vi "GUI_HamamatsuSpectrometer_v1.0.0.vi"() -> ()   [LabVIEW 2013]
uses:
  Shared/MySQL/Preset Query Enum.ctl
  <vilib>/Utility/miscctls.llb/LVOffsetAndMultiplierTypeDef.ctl
  <vilib>/Utility/file.llb/Read From Spreadsheet File (DBL).vi
panel:
  out "FWHM":dbl
  in  "BGlevel":dbl
  out "MeanWavelength":dbl
  out "lambda_r":dbl
  out "lambda_b":dbl
  out "lambda_width (SD)":dbl
  out "AverageCountLevel":dbl
  in  "exposure":dbl
  out "wavelength":dbl[](array[numeric])
  in  "trigger":bool
  in  "save":bool
  out "indecator ref array":refnum<vi>[](array[refnum])
  in  "time to wait (TCP) 2":i32=10
  in  "plot":bool=TRUE
  out "ratio(h)":bool
  out "fixsize":bool
  in  "shotnumber":i32
  out "error (h)":bool
  out "Device Name (h)":string="StagingDG645 1"
  in  "Main Tap":T1(tab)
  out "XY Graph":cluster{"Value":dbl[], "Value":dbl[]}[](graph)
  out "counts":dbl[](array[numeric])
  out "device status::1":string caption="test status"
  out "Intensity Graph 6":dbl[][](graph)
  out "local Port":u16=65427
  out "port or service name":u16=65426
  out "Remote Host":string="192.168.11.97"
  in  "timeout ms (slow resp)":i32=500
  in  "reset":bool
  out "image con closed":bool
  out "image \nconnection":bool
  out "image con closed 2":bool=TRUE
  out "All Devices (h)":string[](array[string])=["StagingDG645 1", "StagingDG645 2"]
  in  "time to wait (TCP)":i32=10
  out "error out":errorcluster
  out "connections (hidden)":variant[](array[variant])=[variant(refnum<k16> refnum), variant(refnum<k16> refnum)]
  in  "time to wait (main loop)":i32=10
  out "Data String":string="Amplitude.Ch AB,3.000000000000\r\nAmplitude.Ch CD,4.000000000000\r\nAmplitude.Ch EF,4.000000000000\r\nAmplitude.Ch GH,4.000000000000\r\nAmplitude.Ch T0,4.000000000000\r\nDelay.Ch A,0.000000000000\r\nDelay.Ch B,0.030000000000\r\nDelay.Ch C,0.000000000000\r\nDelay.Ch D,0.030000000000\r\nDelay.Ch E,0.000000000000\r\nDelay.Ch F,0.030000000000\r\nDelay.Ch G,0.000000000000\r\nDelay.Ch H,0.030000000000\r\nDelay.Ch T0,0.000000000000\r\nDelay.Ch T1,0.030000\r\nInhibit,Triggers\r\nLinked.Ch A,T0\r\nLinked.Ch B,A\r\nLinked.Ch C,T0\r\nLinked.Ch D,C\r\nLinked.Ch E,T0\r\nLinked.Ch F,E\r\nLinked.Ch G,T0\r\nLinked.Ch H,G\r\nLocalSavingPath,c:\\temp\r\nSave,off\r\nTrigger.ExecuteSingleShot,\r\nTrigger.Level,1.000000\r\nTrigger.Rate,10.000000\r\nTrigger.Source,External rising edges\r\ntimeout,0.000000\r\nPolarity.Ch AB,Positive\r\nPolarity.Ch CD,Positive\r\nPolarity.Ch EF,Positive\r\nPolarity.Ch GH,Positive\r\nPolarity.Ch T0,Positive\r\n"
  in  "Local Saving Path":path
  out "error message":string
  out "Data Connection out":bool=TRUE
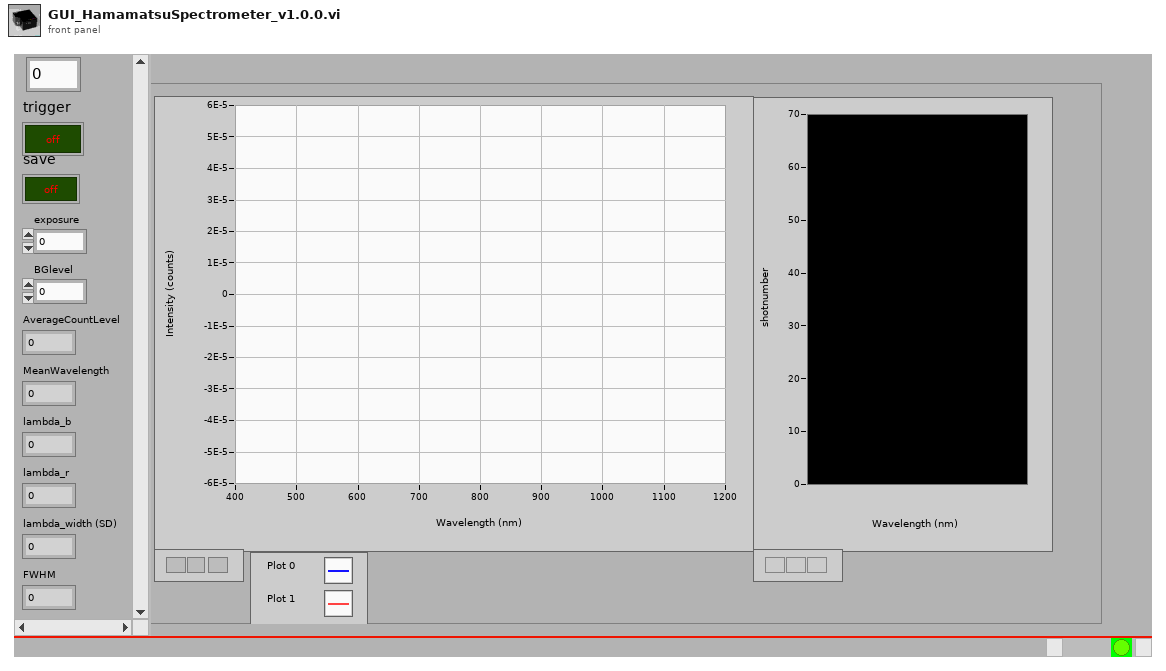
[diagram p1: front panel]
types:
  T1 = enum32{"All Channels", "Network", "Internal", "Advanced"}
  T2 = typedef "Preset Query Enum.ctl" = enum16{"Get Locations", "Get all IPs and MACs", "Get classes", "Get expt variables to set at scanstart for particular device", "Get expt devices and variables with start values", "Get expt devices and variables (with data to get)", "Get expt devices with data to get", "Get Expt devices and GUIs", "Get all devices basic properties", "Get Virtual Devices Core Info", "Get Expt names", "Get experiment basic properties", "Get experiment alarm variables", "Get MC Ports", "Get device network comm port", "Get devicetype lvclass path", "Get basic device properties", "Get Init Order", "Get all setable variables of a device", "Get device variable aliases", "Get force values of all settable variables", "Get all variables of a devicetype", "Get all variables of a device", "Get plotter details", "Get Saved Scans", "Get Scan Info", "GetGeneralGUIs", "Get expt for plotter", "Get plotter IDs from expt", "Get all devices", "Get all Virtual Devices", "Get all aliases", "Get variable and device info for Virtual Device", "GetItemLocatorIP", "Get IPs for GUIs", "Get DeviceType from Device", "GetLocalPortRange", "GetDevicePresetVariables", "Get Device Configuration", "GetAllPresetNames", "GetAllConfigurationNames", "GetPresetDeviceNames"}
  T3 = typedef "LVOffsetAndMultiplierTypeDef.ctl" = cluster{"Offset":dbl, "Multiplier":dbl}
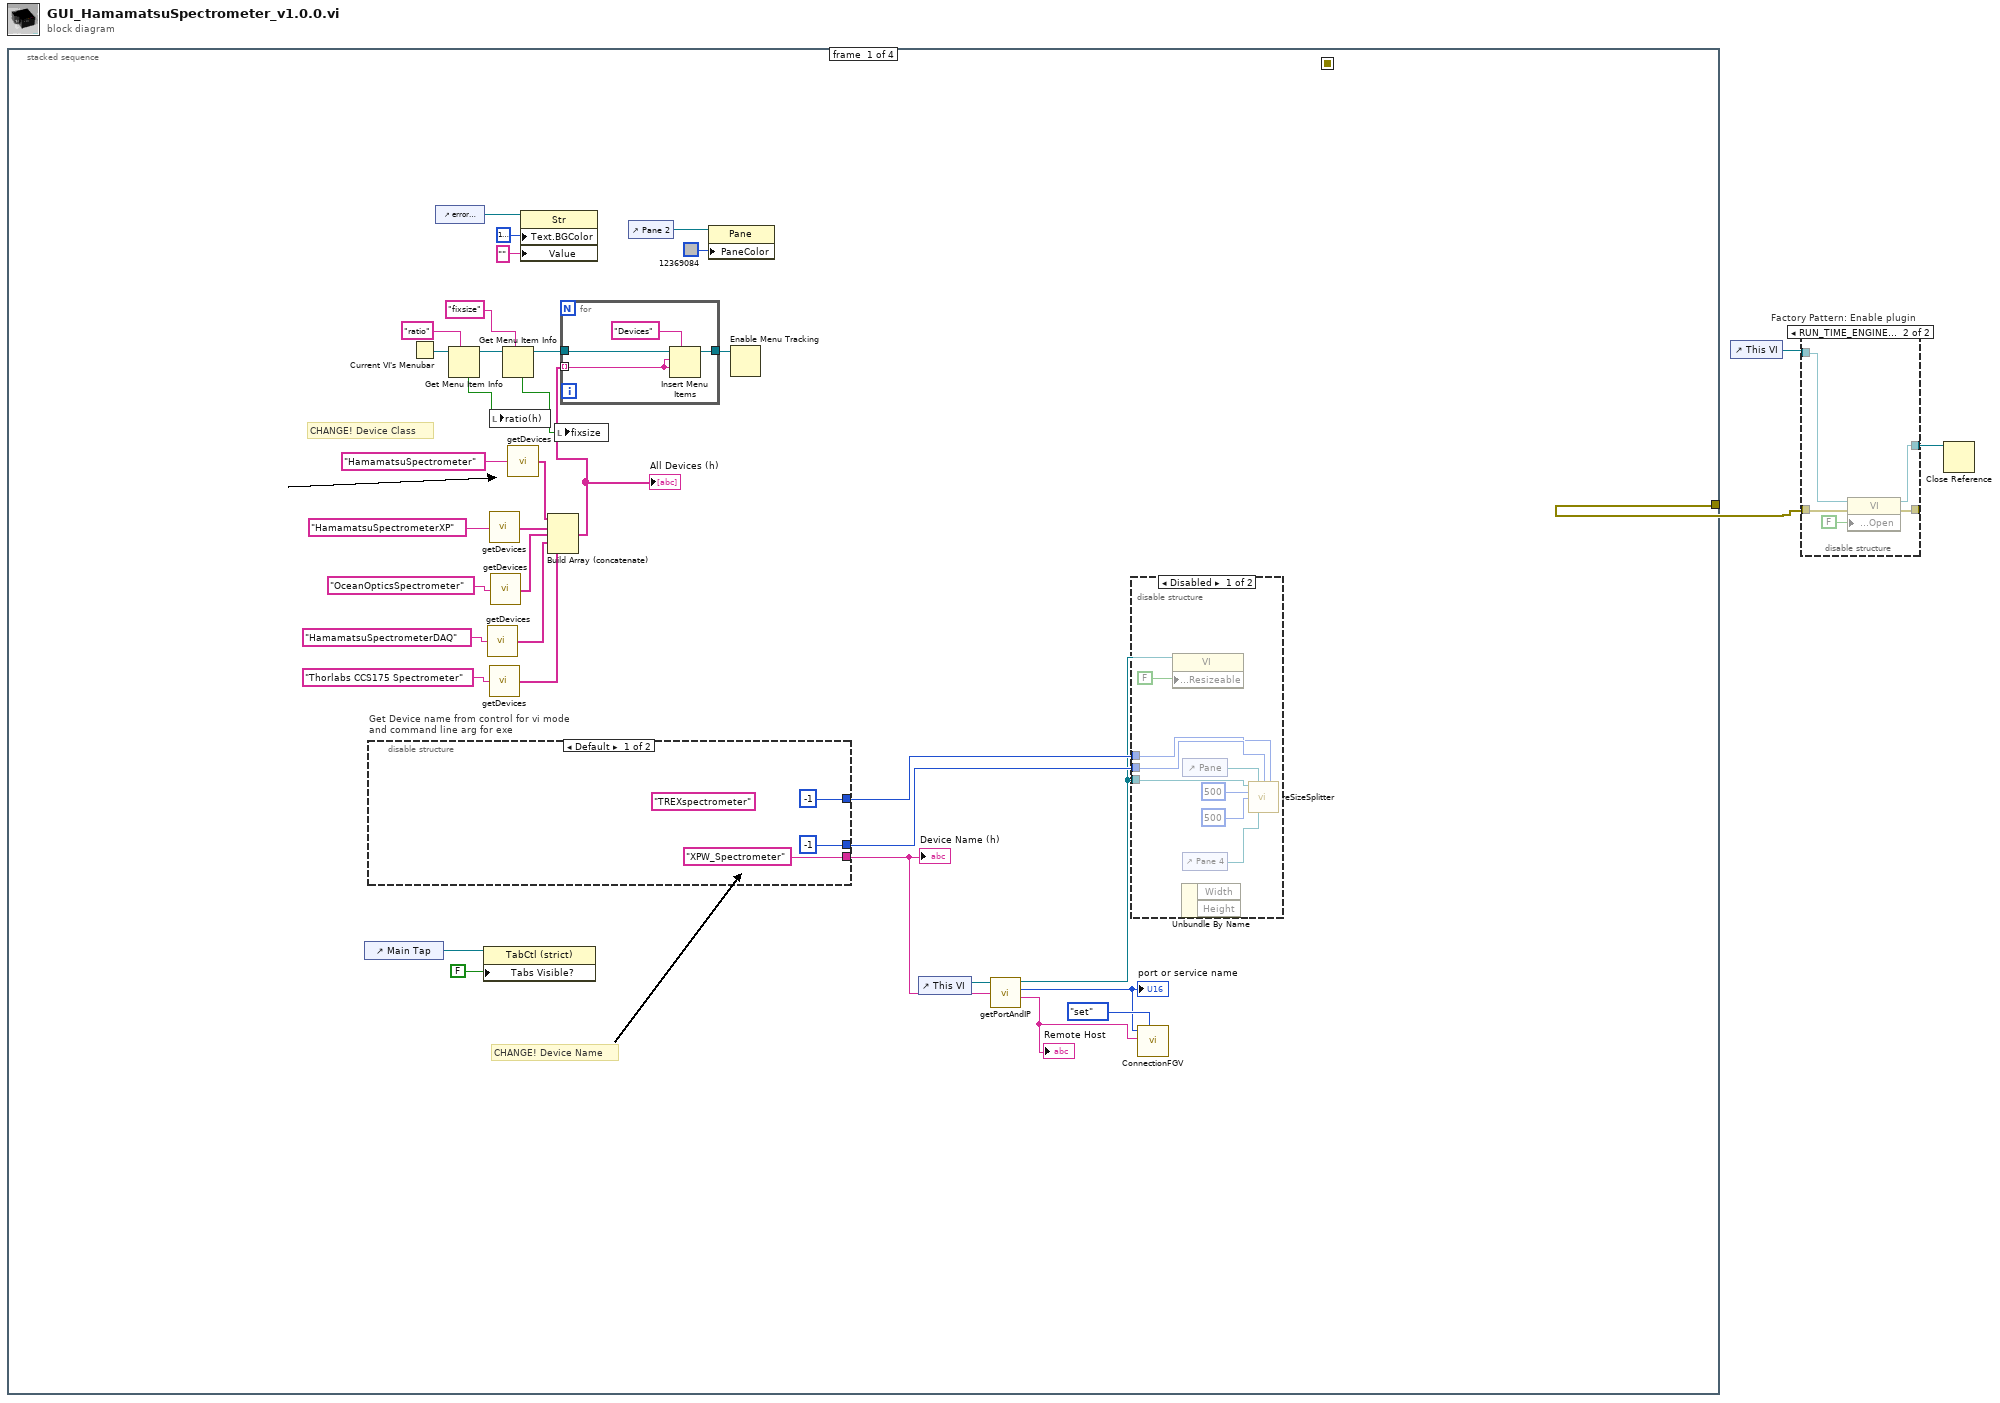
[diagram p0: block diagram]
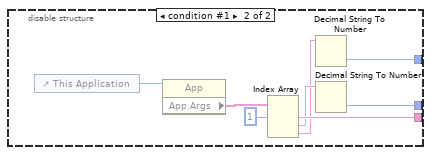
[diagram p4: hidden frame]
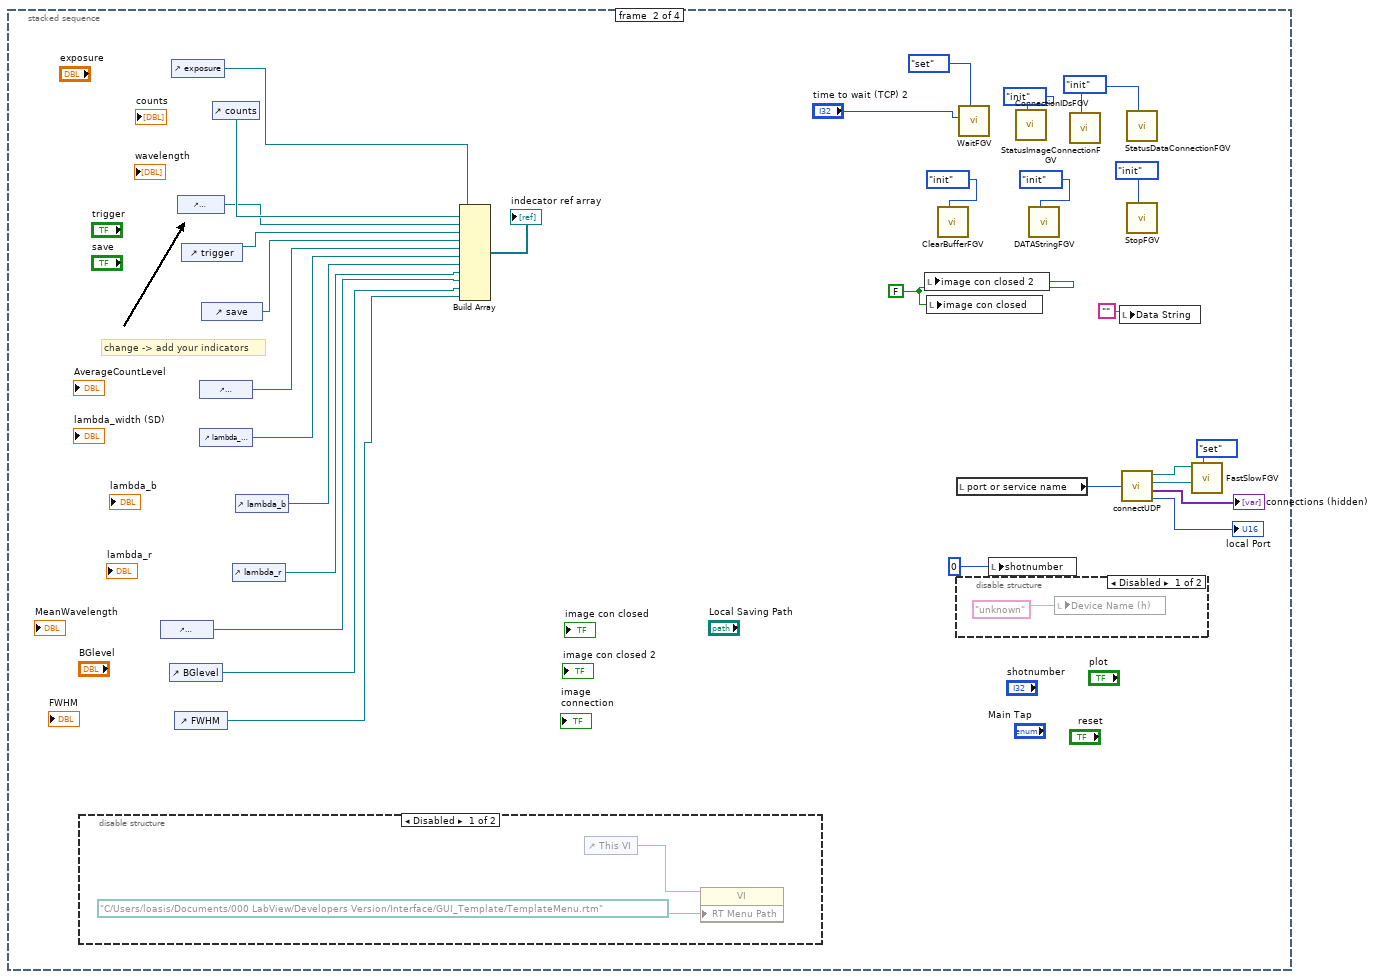
[diagram p5: hidden frame]
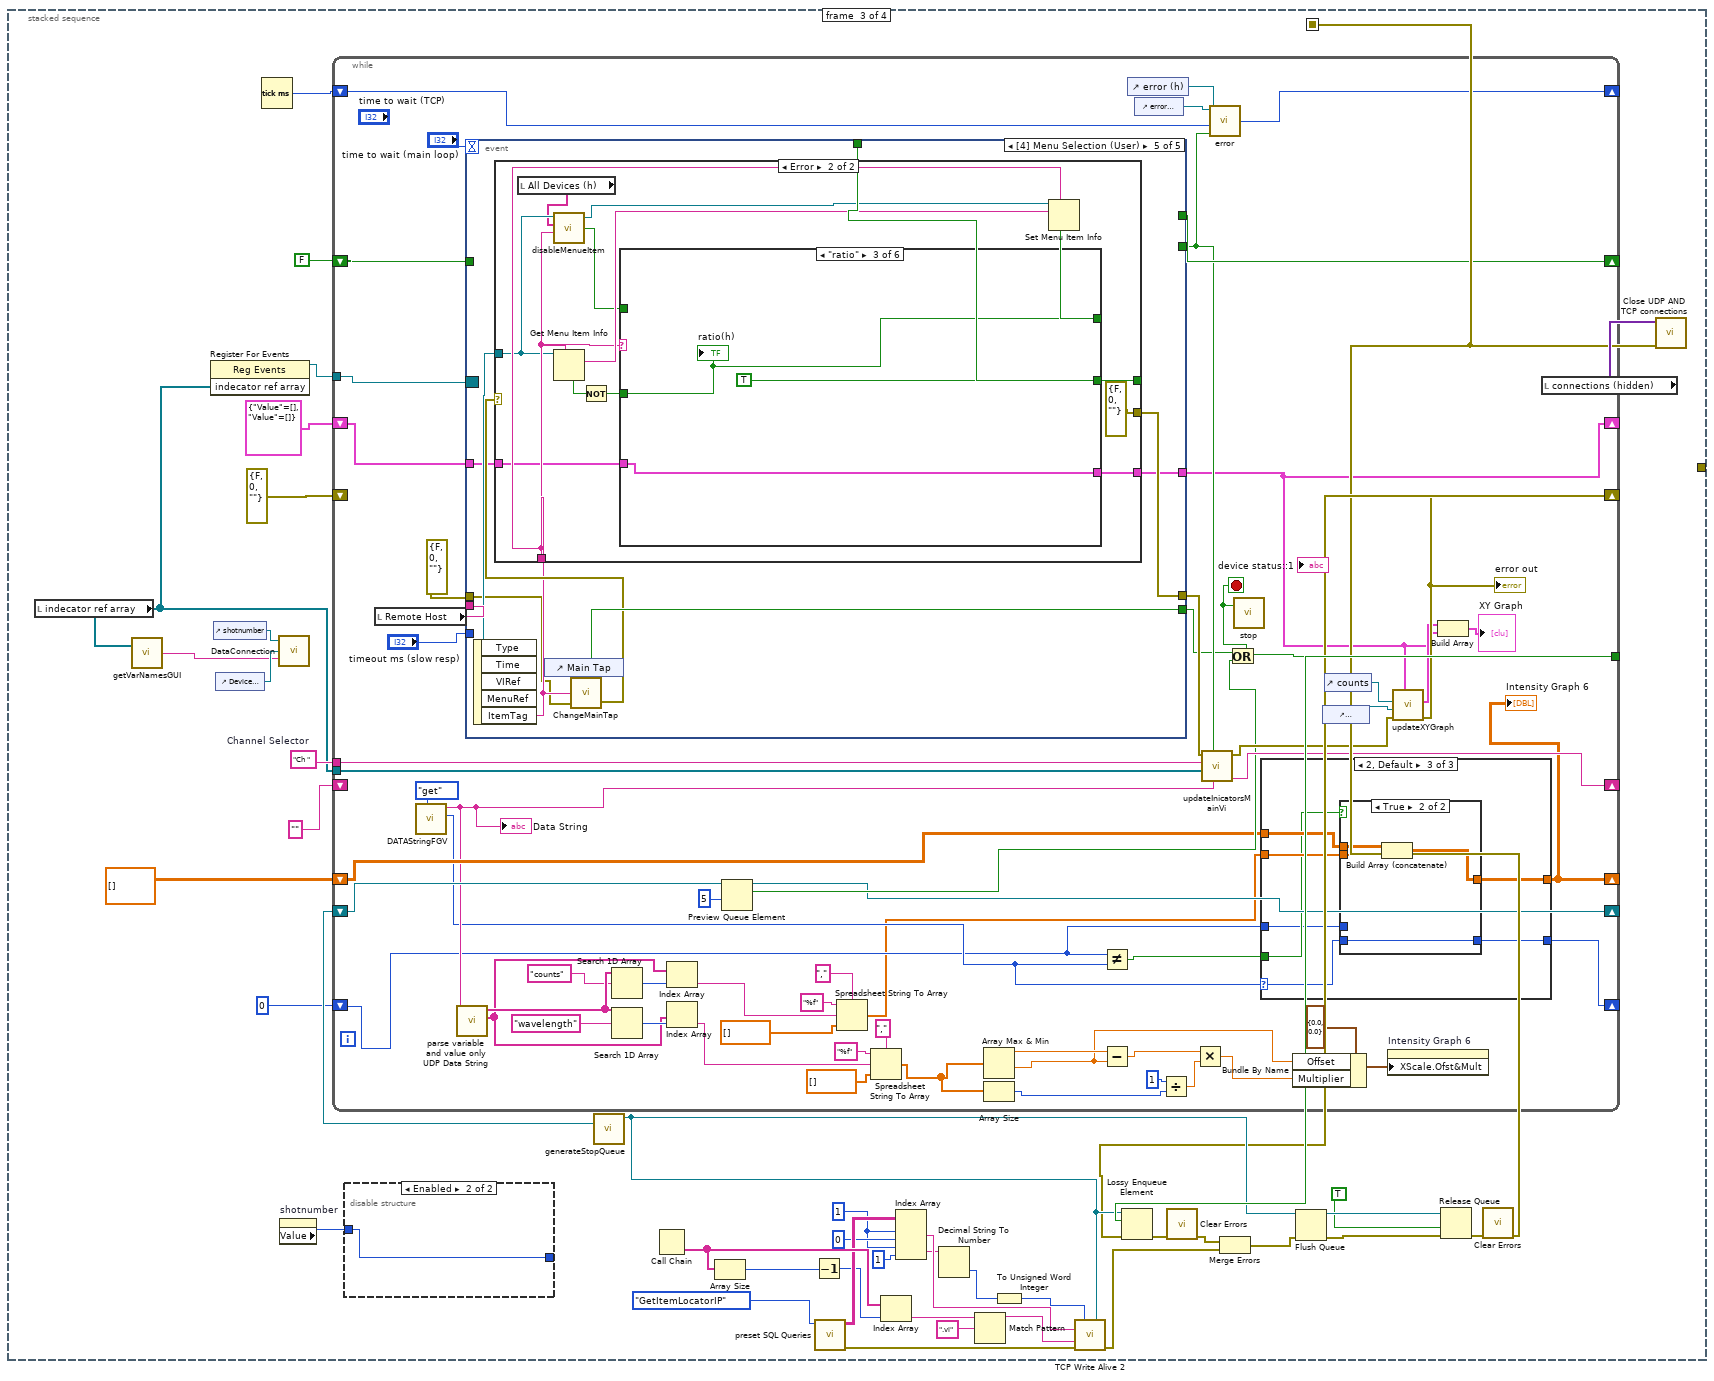
[diagram p8: hidden frame]
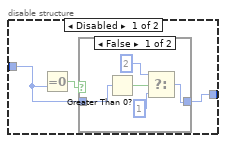
[diagram p9: hidden frame]
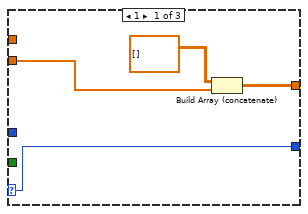
[diagram p11: hidden frame]
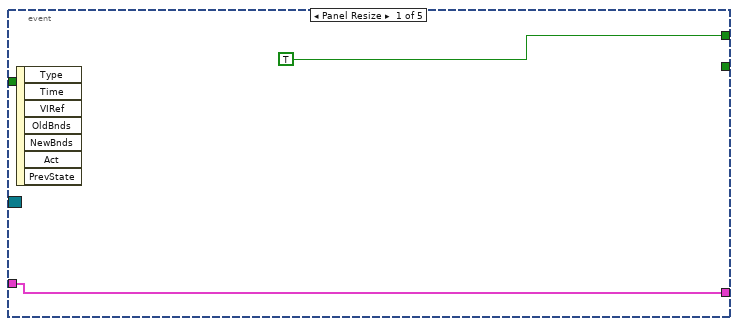
[diagram p14: hidden frame]
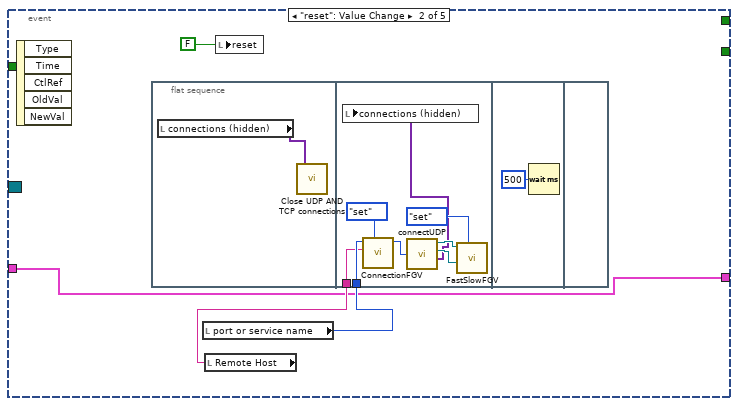
[diagram p15: hidden frame]
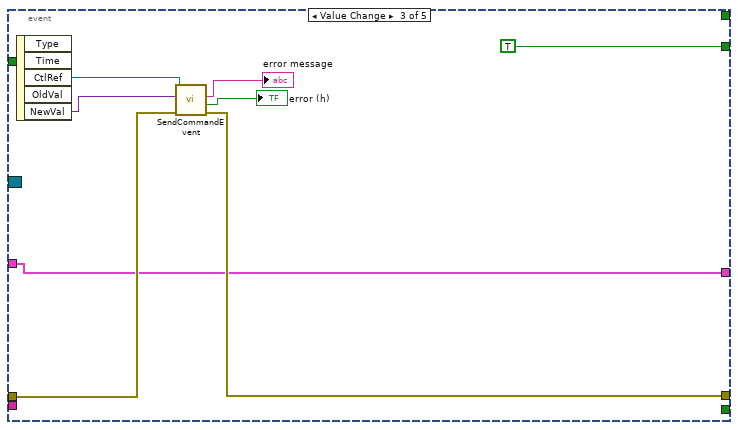
[diagram p16: hidden frame]
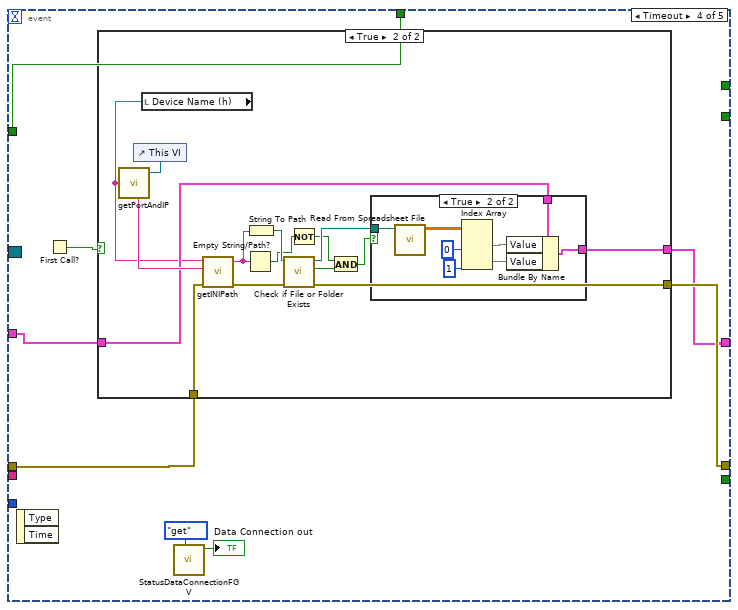
[diagram p17: hidden frame]
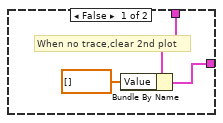
[diagram p19: hidden frame]
diagram:
  n1 = stacked-sequence {
    seq-local: [_ _ w97 _] -> [_ _ _ w368]
    tunnel: [_ _ _ w368] -> w1
    frame #0 {
      # "CHANGE! Device Name"
      # "CHANGE! Device Class"
      n2 = control-ref of="Main Tap"() -> (w38:refnum<vi>)
      n3 = disable-structure "Get Device name from control for vi mode\nand command line arg for exe" shown="Default" {
        disable-tunnel: ["XPW_Spectrometer" ("Device Name for vi mode") w57] -> w34
        disable-tunnel: [i16 -1 ("left") w54] -> w36
        disable-tunnel: [i16 -1 ("left") w53] -> w35
        frame condition #0 (active) {
          (unwired) "TREXspectrometer" ("Device Name for vi mode")
        }
        frame condition #1 {
          n4 = control-ref of="This Application"() -> (w60:refnum<vi>)
          n5 = property class="App"(reference=w60) -> ("App.Args"=w59:string[])  [unwired: 1 in, 2 out]
          n6 = Index Array(array=w59, index #1=1 ("index")) -> (element #1=w57:string, element #2=w56:string, element #3=w55:string)  [unwired: 2 in]
          n7 = Decimal String To Number(string=w55) -> (number=w53:i32)  [unwired: 2 in, 1 out]
          n8 = Decimal String To Number(string=w56) -> (number=w54:i32)  [unwired: 2 in, 1 out]
        }
      }
      "Device Name (h)" <- w34
      n9 = Current VI's Menubar() -> (w26:refnum<k9>)
      n10 = control-ref of="error message"() -> (w20:refnum<vi>)
      n11 = Get Menu Item Info(7:"ratio" ("item tag"), 11:w26) -> (3:w24:refnum<k9>, 4:w25:bool)  [unwired: 1 in, 5 out]
      n12 = property class="TabCtl (strict)"(reference=w38, "Tabs Visible?"=FALSE) -> ()  [unwired: 1 in, 2 out]
      n13 = call "getDevices.vi"("Device Class"="HamamatsuSpectrometerDAQ") -> ("All Devices"=w6:string[])
      n14 = local write "ratio(h)"(w25) -> ()
      n15 = call "getDevices.vi"("Device Class"="HamamatsuSpectrometerXP") -> ("All Devices"=w12:string[])
      n16 = call "getDevices.vi"("Device Class"="Thorlabs CCS175 Spectrometer") -> ("All Devices"=w4:string[])
      n17 = call "getDevices.vi"("Device Class"="OceanOpticsSpectrometer") -> ("All Devices"=w9:string[])
      n18 = Get Menu Item Info(7:"fixsize" ("item tag"), 11:w24) -> (3:w16:refnum<k9>, 4:w22:bool)  [unwired: 1 in, 5 out]
      n19 = call "getDevices.vi"("Device Class"="HamamatsuSpectrometer") -> ("All Devices"=w11:string[])
      n20 = property class="Str"(reference=w20, "Text.BGColor"=u32 16777238, "Value"="") -> ()  [unwired: 1 in, 2 out]
      n21 = Build Array (concatenate)(w11, w12, w9, w6, w4) -> (w10:string[])
      "All Devices (h)" <- w10
      n22 = local write "fixsize"(w22) -> ()
      n23 = for {
        tunnel: w16 -> [w42]
        tunnel: [w41] -> w15
        tunnel: w10 -> [w39] mode=indexing
        n24 = Insert Menu Items(5:"Devices" ("menu tag"), 7:w39, 8:w39, 9:w42) -> (3:w41:refnum<k9>)  [unwired: 2 in, 2 out]
      }
      n25 = control-ref of="Pane 2"() -> (w18:refnum<vi>)
      n26 = property class="Pane"(reference=w18, "PaneColor"=u32 12369084) -> ()  [unwired: 1 in, 2 out]
      n27 = Enable Menu Tracking(4:w15) -> ()  [unwired: 2 in, 2 out]
      n28 = control-ref of="This VI"() -> (w33:refnum<vi>)
      n29 = call "getPortAndIP.vi"("Device Name"=w34, "This Vi"=w33) -> ("Remote Host"=w29:string, "port or service name"=w28:u16, "reference out"=w31:refnum<vi>)  [unwired: 2 in, 2 out]
      "port or service name" <- w28
      "Remote Host" <- w29
      n30 = disable-structure shown="Disabled" {
        disable-tunnel: w36 -> [w48 _]
        disable-tunnel: w35 -> [w47 _]
        disable-tunnel: w31 -> [w45 _]
        frame Disabled {
          n31 = Unbundle By Name() -> ()  [unwired: 1 in, 2 out]
          n32 = control-ref of="Pane"() -> (w49:refnum<vi>)
          n33 = control-ref of="Pane 4"() -> (w46:refnum<vi>)
          n34 = call "reSizeSplitter.vi"("this vi"=w45, "pane"=w49, "left"=w48, "top"=w47, "Width"=u32 500, "Height"=u32 500, "pane2"=w46) -> ()  [unwired: 8 in, 1 out]
        }
        frame Enabled {
        }
      }
      n35 = call "ConnectionFGV.vi"("command"=enum16{"get", "set", "init"}."set", "Remote Host in"=w29, "port or service name in"=w28) -> ()  [unwired: 7 in, 2 out]
      n36 = property class="VI"(reference=w31, "Front Panel.Resizeable"=FALSE ("Front Panel Window:Resizable")) -> ()  [unwired: 1 in, 2 out]
    }
    frame #1 {
      w82 = enum16{"get", "set", "init"}."init" ("Command")
      w88 = FALSE ("new Device Data")
      # "change -> add your indicators"
      n37 = disable-structure shown="Disabled" {
        frame Disabled {
          n38 = control-ref of="This VI"() -> (w92:refnum<vi>)
          n39 = property class="VI"(reference=w92, "RT Menu Path"=path "C:/Users/loasis/Documents/000 LabView/Developers Version/Interface/GUI_Template/TemplateMenu.rtm" ("Run-Time Menu Path")) -> ()  [unwired: 1 in, 2 out]
        }
        frame Enabled {
        }
      }
      n40 = control-ref of="MeanWavelength"() -> (w63:refnum<vi>)
      n41 = control-ref of="BGlevel"() -> (w62:refnum<vi>)
      n42 = control-ref of="exposure"() -> (w68:refnum<vi>)
      n43 = control-ref of="FWHM"() -> (w61:refnum<vi>)
      n44 = control-ref of="wavelength"() -> (w71:refnum<vi>)
      n45 = control-ref of="trigger"() -> (w70:refnum<vi>)
      n46 = control-ref of="AverageCountLevel"() -> (w67:refnum<vi>)
      n47 = control-ref of="lambda_width (SD)"() -> (w66:refnum<vi>)
      n48 = control-ref of="save"() -> (w69:refnum<vi>)
      n49 = control-ref of="counts"() -> (w72:refnum<vi>)
      n50 = control-ref of="lambda_r"() -> (w64:refnum<vi>)
      n51 = control-ref of="lambda_b"() -> (w65:refnum<vi>)
      n52 = Build Array(w68, w72, w71, w70, w69, w67, w66, w65, w64, w63, w62, w61) -> (→"indecator ref array":refnum<vi>[])
      n53 = local write "image con closed 2"(w88) -> ()
      n54 = local write "image con closed"(w88) -> ()
      n55 = call "ClearBufferFGV.vi"("Command"=enum16{"set", "get", "init"}."init") -> ()  [unwired: 10 in, 1 out]
      n56 = local read "port or service name"() -> (w78:u16)
      n57 = disable-structure shown="Disabled" {
        frame Disabled {
          n58 = local write "Device Name (h)"("unknown" ("Device Name")) -> ()
        }
        frame Enabled {
        }
      }
      n59 = call "WaitFGV.vi"("Command"=enum16{"get", "set", "init"}."set", "milliseconds to wait"="time to wait (TCP) 2") -> ()  [unwired: 9 in, 1 out]
      n60 = local write "shotnumber"(0 ("shotnumber")) -> ()
      n61 = call "ConnectionIDsFGV.vi"("Command"=enum16{"add", "get", "init"}."init") -> ()  [unwired: 10 in, 1 out]
      n62 = call "DATAStringFGV.vi"("Command"=enum16{"get", "set", "init"}."init") -> ()  [unwired: 9 in, 2 out]
      n63 = call "StatusImageConnectionFGV.vi"("Command"=w82) -> ()  [unwired: 10 in, 1 out]
      n64 = local write "Data String"("") -> ()
      n65 = call "connectUDP.vi"("port or service name NOT USED"=w78) -> ("fast ID (h)"=w77:refnum<k16>, "slow ID (h)"=w76:refnum<k16>, "connections (hidden)"=→"connections (hidden)":variant[], "local Port"=→"local Port":u16)
      n66 = call "StatusDataConnectionFGV.vi"("Command"=w82) -> ()  [unwired: 10 in, 1 out]
      n67 = call "StopFGV.vi"("Command"=enum16{"set", "get", "init"}."init") -> ()  [unwired: 9 in, 2 out]
      n68 = call "FastSlowFGV.vi"("Command"=enum16{"get", "set", "init"}."set", "slow ID"=w76, "fast ID"=w77) -> ()  [unwired: 7 in, 2 out]
    }
    frame #2 {
      w118 = 1 ("index (row)")
      w127 = "Ch "  # Channel Selector
      n69 = local read "indecator ref array"() -> (w125:refnum<vi>[])
      n70 = call "getVarNamesGUI.vi"("Array"=w125) -> ("String"=w126:string)  [unwired: 1 in]
      n71 = register-events(w125) -> (reference out=w128:refnum<event-registration>)  [unwired: 2 in, 1 out]
      n72 = control-ref of="shotnumber"() -> (w130:refnum<vi>)
      n73 = control-ref of="Device Name (h)"() -> (w129:refnum<vi>)
      n74 = Tick Count (ms)() -> (millisecond timer value=w132:u32)
      n75 = call "DataConnection.vi"("Subscriber list"=w126, "Device Name (h)"=w129, "shotnumber"=w130) -> ()
      n76 = property on="shotnumber" class="DigNum (strict)"() -> ("Value"=w94:i32)  [unwired: 2 in, 2 out]
      n77 = disable-structure shown="Enabled" {
        disable-tunnel: w94 -> [w137 w145]
        disable-tunnel: [w136 w145] -> _
        frame Disabled {
          n78 = Equal To 0?(x=w137) -> (x = 0?=w138:bool)
          n79 = case shown="False" w138 {
            tunnel: w137 -> [w143 w144]
            tunnel: [w139 w144] -> w136
            frame False {
              n80 = Greater Than 0?(x=w143) -> (x > 0?=w142:bool)
              n81 = Select(t=i8 2, s=w142, f=i8 1) -> (s? t:f=w139:i8)
            }
            frame True {
            }
          }
        }
        frame Enabled {
        }
      }
      n82 = call "generateStopQueue.vi"() -> ("STOP Queue out"=w100:refnum<queue>)  [unwired: 10 in, 1 out]
      n83 = while {
        shift-right: [w190] -> w98
        shift-left: errorcluster {"status"=FALSE, "code"=0, "source"=""} ("error out") -> [_]
        tunnel: w125 -> [w199]
        shift-right: [w203] -> _
        shift-left: FALSE -> [w204]
        shift-right: [w202] -> _
        shift-left: w132 -> [w201]
        shift-right: [w194] -> _
        shift-left: "" ("Data String") -> [_]
        tunnel: w128 -> [w197]
        tunnel: w127 -> [w196]
        shift-right: [w184] -> _
        shift-left: w100 -> [w188]
        tunnel: [w185] -> w101
        shift-right: [w182] -> _
        shift-left: dbl[][] [] ("wavelength 2") -> [w183]
        shift-right: [w152] -> _
        shift-left: 0 ("Shot Number") -> [w151]
        shift-right: [w147] -> _
        shift-left: cluster{"Value":dbl[], "Value":dbl[]} {"Value"=[], "Value"=[]} ("reference plot") -> [w149]
        stop <- w185 stop-if-true
        n84 = local read "Remote Host"() -> (w206:string)
        n85 = call "DATAStringFGV.vi"("Command"=enum16{"get", "set", "init"}."get") -> ("Shot Number out"=w154:i32, "Data String out"=w181:string)  [unwired: 9 in]
        "Data String" <- w181
        n86 = call "parse variable and value only UDP Data String.vi"("input string"=w181) -> ("variable values"=w175:string[], "variable names"=w177:string[])  [unwired: 9 in]
        n87 = event shown="[4] Menu Selection (User)" {
          selector: w197 -> [_ _ _ _ _]
          dyn-events: _ -> [_ _ _ _ _]
          timeout: "time to wait (main loop)" -> [_ _ _ _ _]
          tunnel: [_ _ w249 w255 w290] -> w205
          tunnel: w206 -> [_ _ _ _ _]
          tunnel: "timeout ms (slow resp)" -> [_ _ _ _ _]
          tunnel: errorcluster {"status"=FALSE, "code"=0, "source"=""} ("error out") -> [_ _ w246 w256 w291]
          tunnel: [_ _ TRUE _ _] -> w200
          tunnel: [_ _ _ _ w296] -> w187
          tunnel: [_ _ _ w259 w293] -> _
          tunnel: w204 -> [_ _ _ w259 _]
          tunnel: [TRUE _ _ _ _] -> w203
          tunnel: w149 -> [w228 w230 w244 w254 w288]
          tunnel: [w228 w230 w244 w253 w287] -> w147
          event Panel Resize {
            n88 = event-data() -> ()  [unwired: 1 in, 7 out]
          }
          event "reset": Value Change {
            n89 = event-data() -> ()  [unwired: 1 in, 5 out]
            n90 = flat-sequence {
              tunnel: w232 -> [w237]
              tunnel: w231 -> [w236]
              frame #0 {
                n91 = local read "connections (hidden)"() -> (w234:variant[])
                n92 = call "Close UDP AND TCP connections.vi"("appended array"=w234) -> ()  [unwired: 7 in]
              }
              frame #1 {
                n93 = call "ConnectionFGV.vi"("command"=enum16{"get", "set", "init"}."set", "Remote Host in"=w236, "port or service name in"=w237) -> ("port or service name out"=w241:u16)  [unwired: 7 in, 1 out]
                n94 = call "connectUDP.vi"("port or service name NOT USED"=w241) -> ("fast ID (h)"=w240:refnum<k16>, "slow ID (h)"=w239:refnum<k16>, "connections (hidden)"=w235:variant[])  [unwired: 1 out]
                n95 = local write "connections (hidden)"(w235) -> ()
                n96 = call "FastSlowFGV.vi"("Command"=enum16{"get", "set", "init"}."set", "slow ID"=w239, "fast ID"=w240) -> ()  [unwired: 7 in, 2 out]
              }
              frame #2 {
                n97 = Wait (ms)(milliseconds to wait=u32 500) -> ()  [unwired: 1 out]
              }
              frame #3 {
              }
            }
            n98 = local read "port or service name"() -> (w232:u16)
            n99 = local read "Remote Host"() -> (w231:string)
            n100 = local write "reset"(FALSE ("reset")) -> ()
          }
          event Value Change {
            n101 = event-data() -> ("CtlRef"=w251:refnum<vi>, "NewVal"=w250:variant)  [unwired: 1 in, 3 out]
            n102 = call "SendCommandEvent.vi"("error out 2"=w246, "NewVal"=w250, "CtlRef"=w251) -> ("error out"=w249:errorcluster, "error (h)"=→"error (h)":bool, "error message"=→"error message":string)  [unwired: 5 in, 1 out]
          }
          event Timeout {
            n103 = event-data() -> ()  [unwired: 1 in, 2 out]
            n104 = First Call?() -> (First Call?: T/F=w252:bool)
            n105 = case shown="True" w252 {
              tunnel: w256 -> [w260 w266]
              tunnel: [w260 w265] -> w255
              tunnel: w254 -> [w261 w264]
              tunnel: [w261 w263] -> w253
              frame False {
              }
              frame True {
                n106 = control-ref of="This VI"() -> (w275:refnum<vi>)
                n107 = local read "Device Name (h)"() -> (w262:string)
                n108 = call "getPortAndIP.vi"("Device Name"=w262, "This Vi"=w275) -> ("Device Type"=w267:string)  [unwired: 2 in, 4 out]
                n109 = call "getINIPath.vi"("error in (no error)"=w266, "DeviceType Name"=w267, "Device Name"=w262) -> ("error out"=w265:errorcluster, "reference trace path"=w274:string)  [unwired: 7 in]
                n110 = Empty String/Path?(string/path=w274) -> (empty?=w271:bool)
                n111 = String To Path(string=w274) -> (path=w273:path)
                n112 = call <vilib>:"Check if File or Folder Exists.vi"("path"=w273) -> ("file or folder exists?"=w269:bool, "dup path"=w272:path)  [unwired: 8 in, 1 out]
                n113 = Not(x=w271) -> (.not. x?=w270:bool)
                n114 = And(x=w270, y=w269) -> (x .and. y?=w268:bool)
                n115 = case shown="True" w268 {
                  tunnel: w264 -> [w278 w286]
                  tunnel: [w277 w280] -> w263
                  tunnel: w272 -> [_ w279]
                  frame False {
                    # "When no trace,clear 2nd plot"
                    n116 = Bundle By Name(cluster=w278, "Value"=dbl[] []) -> (w277:cluster{"Value":dbl[], "Value":dbl[]})
                  }
                  frame True {
                    n117 = call-poly <vilib>:"Read From Spreadsheet File.vi"("file path (dialog if empty)"=w279) -> ("all rows"=w285:dbl[][])  [unwired: 6 in, 4 out]
                    n118 = Index Array(array=w285, index (col) #1=0 ("disabled index (col)"), index (col) #2=1 ("index (col)")) -> (element #1=w282:dbl[], element #2=w281:dbl[])  [unwired: 2 in]
                    n119 = Bundle By Name(cluster=w286, "Value"=w282, "Value"=w281) -> (w280:cluster{"Value":dbl[], "Value":dbl[]})
                  }
                }
              }
            }
            n120 = call "StatusDataConnectionFGV.vi"("Command"=enum16{"get", "set", "init"}."get") -> ("Data Connection out"=→"Data Connection out":bool)  [unwired: 10 in]
          }
          event Menu Selection (User) {
            n121 = event-data() -> ("MenuRef"=w292:refnum<k9>, "ItemTag"=w294:string)  [unwired: 1 in, 3 out]
            n122 = control-ref of="Main Tap"() -> (w289:refnum<vi>)
            n123 = call "ChangeMainTap.vi"("error in"=w291, "ItemTag"=w294, "reference"=w289) -> ("error out"=w295:errorcluster, "Boolean"=w296:bool)
            n124 = case shown="Error" w295 {
              selector: w295 -> [w298 _]
              tunnel: w292 -> [_ w306]
              tunnel: [_ w308] -> w293
              tunnel: w294 -> [_ w307]
              tunnel: [w298 errorcluster {"status"=FALSE, "code"=0, "source"=""} ("error IO")] -> w290
              tunnel: w288 -> [w297 w300]
              tunnel: [w297 w299] -> w287
              frame No Error {
              }
              frame Error {
                n125 = local read "All Devices (h)"() -> (w301:string[])
                n126 = call "disableMenueItem.vi"("ItemTag"=w307, "All Devices (h)"=w301, "MenuRef"=w306) -> ("this is a Device(tag)"=w305:bool, "menu reference out"=w304:refnum<k9>)  [unwired: 1 in, 1 out]
                n127 = Get Menu Item Info(7:w307, 11:w306) -> (2:w310:string, 4:w311:bool)  [unwired: 1 in, 5 out]
                n128 = Not(x=w311) -> (.not. x?=w309:bool)
                n129 = case shown="\"ratio\"" w307 {
                  selector: w307 -> [_ w320 _ _ _ _]
                  tunnel: w309 -> [w313 w318 w352 _ _ _]
                  tunnel: [_ _ TRUE _ _ _] -> w308
                  tunnel: w305 -> [_ w321 _ _ _ _]
                  tunnel: [w313 w319 w352 _ _ _] -> w303
                  tunnel: w300 -> [w312 w317 w351 w354 w362 w365]
                  tunnel: [w312 w316 w351 w354 w362 w365] -> w299
                  frame "fixsize" {
                    n130 = control-ref of="This VI"() -> (w315:refnum<vi>)
                    n131 = Not(x=w313) -> (.not. x?=w314:bool)
                    n132 = property class="VI"(reference=w315, "Front Panel.Resizeable"=w314) -> ()  [unwired: 1 in, 2 out]
                    "fixsize" <- w313
                  }
                  frame Default {
                    n133 = case shown="True" w321 {
                      tunnel: w320 -> [_ w323]
                      tunnel: [_ w334] -> w319
                      tunnel: w318 -> [_ w334]
                      tunnel: w317 -> [w322 w333]
                      tunnel: [w322 w332] -> w316
                      frame False {
                      }
                      frame True {
                        n134 = control-ref of="This VI"() -> (w339:refnum<vi>)
                        n135 = call "getPortAndIP.vi"("Device Name"=w323, "This Vi"=w339) -> ("Device Type"=w331:string, "Remote Host"=w338:string, "port or service name"=w337:u16)  [unwired: 2 in, 2 out]
                        n136 = call "getINIPath.vi"("DeviceType Name"=w331, "Device Name"=w323) -> ("reference trace path"=w330:string)  [unwired: 8 in, 1 out]
                        n137 = local write "Remote Host"(w338) -> ()
                        n138 = local write "port or service name"(w337) -> ()
                        n139 = Empty String/Path?(string/path=w330) -> (empty?=w327:bool)
                        n140 = String To Path(string=w330) -> (path=w329:path)
                        n141 = call <vilib>:"Check if File or Folder Exists.vi"("path"=w329) -> ("file or folder exists?"=w325:bool, "dup path"=w328:path)  [unwired: 8 in, 1 out]
                        n142 = Not(x=w327) -> (.not. x?=w326:bool)
                        n143 = And(x=w326, y=w325) -> (x .and. y?=w324:bool)
                        n144 = control-ref of="reset"() -> (w336:refnum<vi>)
                        n145 = case shown="True" w324 {
                          tunnel: w333 -> [w342 w350]
                          tunnel: [w341 w344] -> w332
                          tunnel: w328 -> [_ w343]
                          frame False {
                            # "When no trace,clear 2nd plot"
                            n146 = Bundle By Name(cluster=w342, "Value"=dbl[] []) -> (w341:cluster{"Value":dbl[], "Value":dbl[]})
                          }
                          frame True {
                            n147 = call-poly <vilib>:"Read From Spreadsheet File.vi"("file path (dialog if empty)"=w343) -> ("all rows"=w349:dbl[][])  [unwired: 6 in, 4 out]
                            n148 = Index Array(array=w349, index (col) #1=0 ("disabled index (col)"), index (col) #2=1 ("index (col)")) -> (element #1=w346:dbl[], element #2=w345:dbl[])  [unwired: 2 in]
                            n149 = Bundle By Name(cluster=w350, "Value"=w346, "Value"=w345) -> (w344:cluster{"Value":dbl[], "Value":dbl[]})
                          }
                        }
                        n150 = property class="Bool (strict)"(reference=w336, "Val(Sgnl)"=TRUE ("Value (Signaling)")) -> ()  [unwired: 1 in, 2 out]
                      }
                    }
                  }
                  frame "ratio" {
                    "ratio(h)" <- w352
                  }
                  frame "Local Saving Path" {
                    n151 = control-ref of="Local Saving Path"() -> (w355:refnum<vi>)
                    n152 = property class="Path"(reference=w355) -> (reference out=w358:refnum<vi>, "Value"=w359:path)  [unwired: 1 in, 1 out]
                    n153 = call "changePath.vi"("Local Saving in (h)"=w359) -> ("change (h)"=w357:bool, "Local Saving out (h)"=w356:path)  [unwired: 9 in]
                    n154 = case shown="True" w357 {
                      tunnel: w358 -> [_ w361]
                      tunnel: w356 -> [_ w360]
                      frame False {
                      }
                      frame True {
                        n155 = property class="Path"(reference=w361, "Val(Sgnl)"=w360) -> ()  [unwired: 1 in, 2 out]
                      }
                    }
                  }
                  frame "reset" {
                    n156 = control-ref of="reset"() -> (w364:refnum<vi>)
                    n157 = property class="Bool (strict)"(reference=w364, "Val(Sgnl)"=TRUE ("Value (Signaling)")) -> ()  [unwired: 1 in, 2 out]
                  }
                  frame "clear" {
                    n158 = control-ref of="reset"() -> (w367:refnum<vi>)
                    n159 = property class="Bool (strict)"(reference=w367, "Val(Sgnl)"=TRUE ("Value (Signaling)")) -> ()  [unwired: 1 in, 2 out]
                  }
                }
                n160 = Set Menu Item Info(6:w303, 7:w307, 10:w310, 11:w304) -> ()  [unwired: 3 in, 2 out]
              }
            }
          }
        }
        n161 = Search 1D Array(1D array=w177, element="counts") -> (index of element=w176:i32)  [unwired: 1 in]
        n162 = Search 1D Array(1D array=w177, element="wavelength") -> (index of element=w179:i32)  [unwired: 1 in]
        n163 = Index Array(array=w175, index=w176) -> (element=w170:string)
        n164 = Index Array(array=w175, index=w179) -> (element=w165:string)
        n165 = Preview Queue Element ("get stop queue value")(queue=w188, timeout in ms (-1)=5) -> (queue out=w184:refnum<queue>, element=w186:bool)  [unwired: 1 in, 2 out]
        n166 = Spreadsheet String To Array(delimiter (Tab)=",", format string="%f", spreadsheet string=w170, array type (2D Dbl)=dbl[] []) -> (array=w150:dbl[])
        n167 = Spreadsheet String To Array(delimiter (Tab)=",", format string="%f", spreadsheet string=w165, array type (2D Dbl)=dbl[] []) -> (array=w164:dbl[])
        n168 = Array Max & Min(array=w164) -> (max value=w161:dbl, min value=w156:dbl)  [unwired: 2 out]
        n169 = Array Size(array=w164) -> (size(s)=w163:i32)
        n170 = Not Equal?(x=w151, y=w154) -> (x != y?=w153:bool)
        n171 = Subtract(x=w161, y=w156) -> (x-y=w160:dbl)
        n172 = control-ref of="error (h)"() -> (w192:refnum<vi>)
        n173 = control-ref of="error message"() -> (w193:refnum<vi>)
        n174 = Divide(x=1, y=w163) -> (x/y=w159:dbl)
        n175 = Multiply(x=w160, y=w159) -> (x*y=w155:dbl)
        n176 = call "updateInicatorsMainVi.vi"("Data String out"=w181, "Boolean"=w200, "Array"=w199, "Channel Selector"=w196, "error in"=w205) -> ("Data String out 2"=w194:string, "error out"=w191:errorcluster)  [unwired: 4 in, 1 out]
        n177 = call "error.vi"("Boolean"=w200, "millisecond timer value"=w201, "reference"=w192, "error message"=w193) -> ("millisecond timer value 2"=w202:u32)
        n178 = Or(x=w187, y=w186) -> (x .or. y?=w185:bool)
        n179 = call "stop.vi"("Boolean"=w185) -> ()
        n180 = case shown="2, Default" w154 {
          selector: w154 -> [w209 w213 w217]
          tunnel: w183 -> [_ w214 w221]
          tunnel: w150 -> [w211 _ w220]
          tunnel: [w210 w214 w219] -> w182
          tunnel: w153 -> [_ _ w218]
          tunnel: [w209 w213 w216] -> w152
          tunnel: w151 -> [_ _ w215]
          frame 1 {
            n181 = Build Array (concatenate)(dbl[][] [] ("wavelength 2"), w211) -> (w210:dbl[][])
          }
          frame 0 {
          }
          frame 2, Default {
            n182 = case shown="True" w218 {
              tunnel: w221 -> [w223 w227]
              tunnel: [w223 w226] -> w219
              tunnel: w220 -> [_ w225]
              tunnel: w217 -> [_ w224]
              tunnel: [w222 w224] -> w216
              tunnel: w215 -> [w222 _]
              frame False {
              }
              frame True {
                n183 = Build Array (concatenate)(w227, w225) -> (w226:dbl[][])
              }
            }
          }
        }
        "Intensity Graph 6" <- w182
        n184 = Bundle By Name(cluster=T3 {"Offset"=0.0, "Multiplier"=0.0} ("X Scale.Offset and Multiplier"), "Offset"=w156, "Multiplier"=w155) -> (w157:T3)
        n185 = control-ref of="wavelength"() -> (w178:refnum<vi>)
        n186 = control-ref of="counts"() -> (w180:refnum<vi>)
        n187 = property on="Intensity Graph 6" class="IntGraph (strict)"("XScale.Ofst&Mult"=w157) -> ()  [unwired: 2 in, 2 out]
        n188 = call "updateXYGraph.vi"("reference plot"=w147, "error in (no error)"=w191, "wavelength"=w178, "counts"=w180) -> ("error out"=w190:errorcluster, "output cluster"=w148:cluster{"Value":dbl[], "Value":dbl[]})  [unwired: 6 in]
        "error out" <- w190
        n189 = Build Array(w148, w147) -> (→"XY Graph":cluster{"Value":dbl[], "Value":dbl[]}[])
      }
      n190 = Call Chain() -> (call chain=w124:string[])
      n191 = Array Size(array=w124) -> (size(s)=w109:i32)
      n192 = Decrement(x=w109) -> (x-1=w110:i32)
      n193 = call "preset SQL Queries.vi"("Preset Query"=Preset_Query_Enum."GetItemLocatorIP") -> ("error out"=w115:errorcluster, "data"=w121:string[][])  [unwired: 8 in, 1 out]
      n194 = Index Array(array=w124, index=w110) -> (element=w111:string)
      n195 = Index Array(array=w121, index (row) #1=w118, index (col) #1=0 ("disabled index (col)"), index (row) #2=w118, index (col) #2=1 ("disabled index (col)")) -> (element #1=w123:string, element #2=w122:string)
      n196 = Decimal String To Number(string=w122) -> (number=w116:i32)  [unwired: 2 in, 1 out]
      n197 = Match Pattern(string=w111, regular expression=".vi") -> (before substring=w113:string)  [unwired: 1 in, 3 out]
      n198 = To Unsigned Word Integer(number=w116) -> (unsigned 16bit integer=w117:u16)
      n199 = call "TCP Write Alive 2.vi"("MultiCast Port"=w117, "Stopqueue"=w100, "address"=w123, "Name"=w113, "error in (no error)"=w115) -> ("error out"=w99:errorcluster)  [unwired: 8 in, 2 out]
      n200 = Lossy Enqueue Element(queue=w100, element=w101, error in (no error)=w98) -> (error out=w102:errorcluster)  [unwired: 3 out]
      n201 = call <vilib>:"Clear Errors.vi"("error in (no error)"=w102) -> ("error out"=w103:errorcluster)  [unwired: 6 in]
      n202 = Merge Errors(w103, w99) -> (w107:errorcluster)
      n203 = Flush Queue(queue=w100, error in (no error)=w107) -> (queue out=w108:refnum<queue>, error out=w104:errorcluster)  [unwired: 1 out]
      n204 = Release Queue(queue=w108, force destroy? (F)=TRUE, error in (no error)=w104) -> (error out=w106:errorcluster)  [unwired: 2 out]
      n205 = call <vilib>:"Clear Errors.vi"("error in (no error)"=w106) -> ("error out"=w97:errorcluster)  [unwired: 6 in]
      n206 = local read "connections (hidden)"() -> (w134:variant[])
      n207 = call "Close UDP AND TCP connections.vi"("error in"=w97, "appended array"=w134) -> ()  [unwired: 6 in]
    }
    frame #3 {
      n208 = control-ref of="Main  Control"() -> (w370:refnum<vi>)
      n209 = property class="TabCtl (strict)"(reference=w370, "Tabs Visible?"=TRUE) -> ()  [unwired: 1 in, 2 out]
      n210 = property class="TabCtl (strict)"(reference=w370, "Tab Location"=enum32{"Top", "Bottom", "Left", "Right"}."Bottom") -> ()  [unwired: 1 in, 2 out]
      n211 = flat-sequence {
        frame #0 {
          n212 = Wait (ms)(milliseconds to wait=u32 0) -> ()  [unwired: 1 out]
        }
        frame #1 {
        }
        frame #2 {
          n213 = disable-structure shown="Disabled" {
            frame Disabled {
              n214 = control-ref of="This VI"() -> (w375:refnum<vi>)
              n215 = case shown="True" FALSE {
                tunnel: w375 -> [w376 w379]
                tunnel: [w376 w377] -> w374
                frame False {
                }
                frame True {
                  n216 = property class="VI" props=["Front Panel.Open"](reference=w379) -> (reference out=w378:refnum<vi>)  [unwired: 1 in, 2 out]
                  n217 = invoke class="VI" method="FP.Close"(reference=w378) -> (reference out=w377:refnum<vi>)  [unwired: 2 in, 2 out]
                }
              }
              n218 = Close Reference(reference=w374) -> ()  [unwired: 1 in, 1 out]
            }
            frame Enabled {
            }
          }
        }
      }
    }
  }
  n219 = control-ref of="This VI"() -> (w2:refnum<vi>)
  n220 = disable-structure "Factory Pattern: Enable plugin" shown="RUN_TIME_ENGINE==True" {
    disable-tunnel: w1 -> [_ w384]
    disable-tunnel: w2 -> [w380 w383]
    disable-tunnel: [_ w382] -> _
    disable-tunnel: [w380 w381] -> w3
    frame condition #0 (active) {
    }
    frame condition #1 {
      n221 = property class="VI"(reference=w383, error in=w384, "Front Panel.Open"=FALSE) -> (reference out=w381:refnum<vi>, error out=w382:errorcluster)
    }
  }
  n222 = Close Reference(reference=w3) -> ()  [unwired: 1 in, 1 out]
